vi "apply data indices.vi"(8 "error in":errorcluster, 10 "index type defs":T1, 11 "Watchdog runtime in":refnum<class "Watchdog runtime.lvclass">) -> (0 "error out":errorcluster, 3 "Watchdog runtime out":refnum<class "Watchdog runtime.lvclass">)   [LabVIEW 2013, in "Watchdog runtime.lvclass"]
uses:
  Watchdog runtime.lvclass
  <vilib>/NI/Tag Bus Data Framework/fixed module parent/module/configuration/index type definitions.ctl
  configuration/input data indices.ctl
  configuration/output data indices.ctl
  configuration/parameter data indices.ctl
  configuration/result data indices.ctl
  Watchdog runtime.lvclass/Watchdog runtime.ctl
  configuration/Watchdog configuration.lvclass
  <vilib>/NI/Tag Bus Data Framework/fixed module parent/module/configuration/fixed channel configuration.lvclass
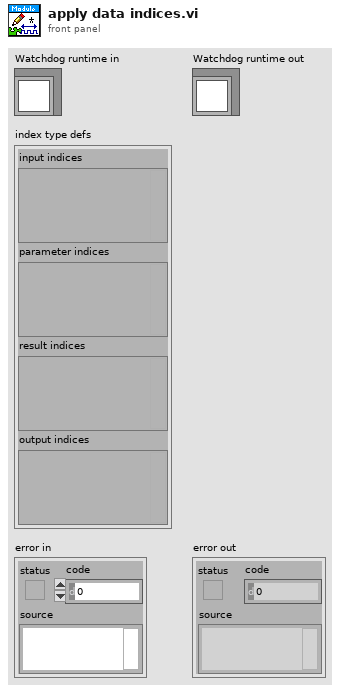
[diagram p1: front panel]
types:
  T1 = typedef "fixed channel configuration.lvclass/index type definitions.ctl" = cluster{"input indices":variant, "parameter indices":variant, "result indices":variant, "output indices":variant}
  T2 = typedef "Watchdog configuration.lvclass/result data indices.ctl" = cluster{"placeholder":i32}
  T3 = typedef "Watchdog configuration.lvclass/parameter data indices.ctl" = cluster{"U8.counter":i32}
  T4 = typedef "Watchdog configuration.lvclass/output data indices.ctl" = cluster{"placeholder":i32}
  T5 = typedef "Watchdog configuration.lvclass/input data indices.ctl" = cluster{"placeholder":i32}
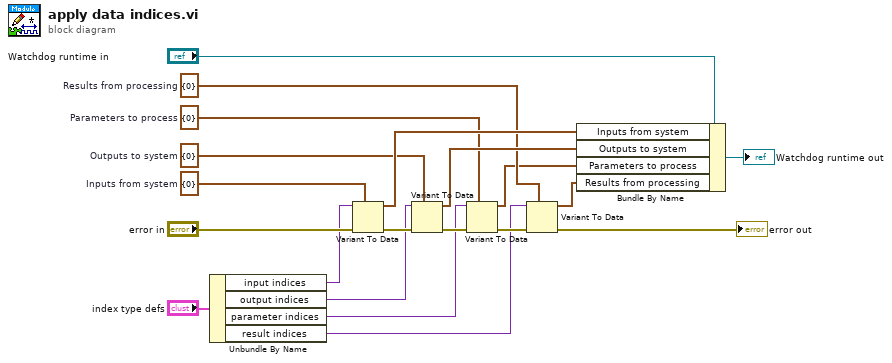
[diagram p0: block diagram]
diagram:
  w3 = T2 {"placeholder"=0}  # Results from processing
  w4 = T3 {"U8.counter"=0}  # Parameters to process
  w8 = T4 {"placeholder"=0}  # Outputs to system
  w11 = T5 {"placeholder"=0}  # Inputs from system
  n1 = Unbundle By Name("index type defs") -> ("input indices"=w12:variant, "output indices"=w9:variant, "parameter indices"=w6:variant, "result indices"=w5:variant)
  n2 = Variant To Data(error in="error in", type=w11, Variant=w12) -> (data=w10:T5, error out=w13:errorcluster)
  n3 = Variant To Data(error in=w13, type=w8, Variant=w9) -> (data=w7:T4, error out=w16:errorcluster)
  n4 = Variant To Data(error in=w16, type=w4, Variant=w6) -> (data=w2:T3, error out=w14:errorcluster)
  n5 = Variant To Data(error in=w14, type=w3, Variant=w5) -> (data=w1:T2, error out=→"error out":errorcluster)
  n6 = Bundle By Name(cluster="Watchdog runtime in", "Inputs from system"=w10, "Outputs to system"=w7, "Parameters to process"=w2, "Results from processing"=w1) -> (→"Watchdog runtime out":refnum<class "Watchdog runtime.lvclass">)
